vi "MALT Close.vi"(8 "error in":errorcluster) -> (0 "error out":errorcluster)   [LabVIEW 2018, in "AltonTech MALT200817.lvlib"]
uses:
  <instrlib>/AltonTech MALT/AltonTech MALT200817.lvlib
  <instrlib>/AltonTech MALT/Private/Global/MALT Global.vi
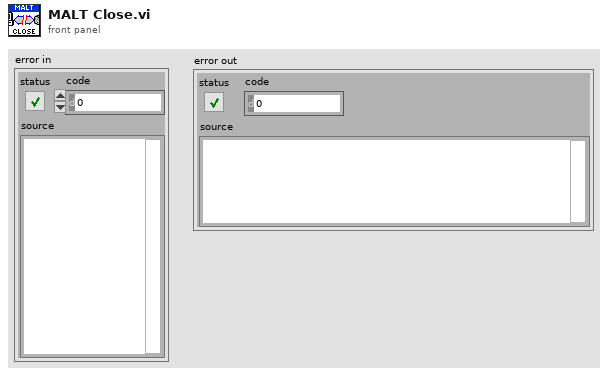
[diagram p1: front panel]
types:
  T1 = cluster{"Timeout":i32, "CAN Response Delay":i32, "Connection ID":refnum<k5>, "config file path":path}
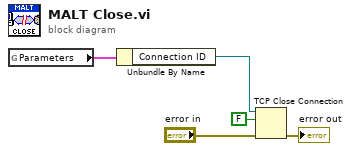
[diagram p0: block diagram]
diagram:
  n1 = global read "MALT Global.vi" "Parameters"() -> (w2:T1)
  n2 = Unbundle By Name(w2) -> ("Connection ID"=w1:refnum<k5>)
  n3 = TCP Close Connection(connection ID=w1, abort (F)=FALSE, error in (no error)="error in") -> (error out=→"error out":errorcluster)  [unwired: 1 out]
